vi "Dev List - New DTRow.vi"(7 "Row Index":i32, 8 "error in (no error)":errorcluster, 9 "Dev Data Lookup Table in":variant, 10 "DataGridView in":refnum<class "DataGridView.lvclass">, 11 "Controller UI in":refnum<class "Controller UI.lvclass">) -> (0 "error out":errorcluster, 1 "Dev Data Lookup Table in out":variant, 2 "DataGridView out":refnum<class "DataGridView.lvclass">)   [LabVIEW 2016, in "Controller UI.lvlib" / "Controller UI.lvclass"]
uses:
  <userlib>/Common Components/Controller UI/Controller UI.lvclass
  <userlib>/LabVIEWdotNetDataGrid/source/DataGridView/DataGridView.lvclass
  <userlib>/Common Components/Hardware/DevInfo/DevInfo Cluster Constant.ctl
  <userlib>/Common Components/Controller UI/Dev Variant Data.ctl
  <userlib>/Common Components/Hardware/DevInfo/DevInfo.lvclass
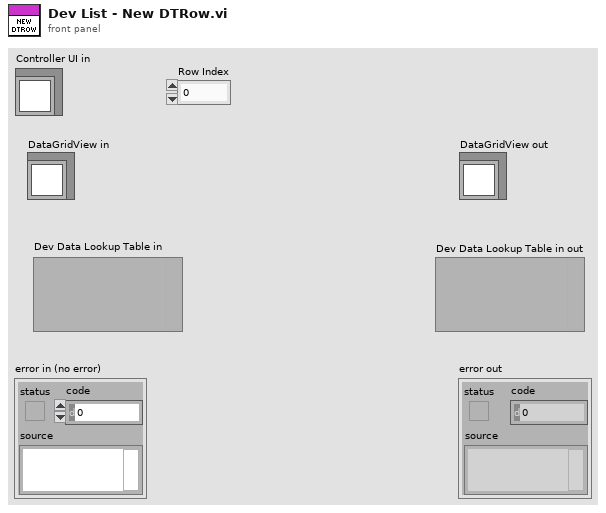
[diagram p1: front panel]
types:
  T1 = typedef "Controller UI.lvlib/Controller UI.lvclass/Dev Variant Data.ctl" = cluster{"Row Index":i32, "DevInfo Obj":refnum<class "DevInfo.lvclass">}
  T2 = typedef "Hardware.lvlib/DevInfo.lvclass/DevInfo Cluster Constant.ctl" = cluster{"GUID":string, "Check":string, "Checked-out":string, "Status":string, "Device":string, "Label":string, "COMM":string, "Sub-COMM":string, "COMM Settings":string}
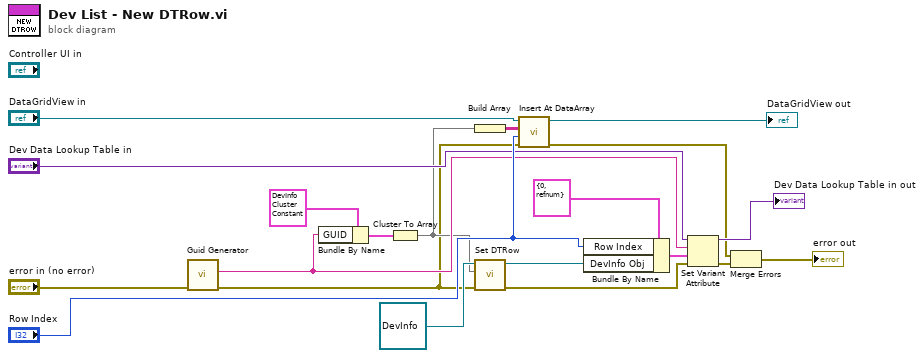
[diagram p0: block diagram]
diagram:
  n1 = call <vilib>:"Guid Generator.vi"("error in (no error)"="error in (no error)") -> ("error out"=w4:errorcluster, "GUID"=w11:string)  [unwired: 9 in]
  n2 = Bundle By Name(cluster=T2 {"GUID"="", "Check"="False", "Checked-out"="False", "Status"="off.png", "Device"="", "Label"="Enter a label", "COMM"="", "Sub-COMM"="", "COMM Settings"=""} ("Cluster"), "GUID"=w11) -> (w12:T2)
  n3 = Cluster To Array(cluster=w12) -> (array=w8:string[])
  n4 = Build Array(w8) -> (w14:string[][])
  n5 = call <userlib>:"Set DTRow.vi"("error in (no error)"=w4, "Dev Row Elements"=w8, "DevInfo in"=refnum<class "DevInfo.lvclass"> refnum ("DevInfo Obj")) -> ("error out"=w3:errorcluster, "DevInfo out"=w7:refnum<class "DevInfo.lvclass">)  [unwired: 7 in]
  n6 = call <userlib>:"Insert At DataArray.vi"("error in"=w4, "index"="Row Index", "Rows"=w14, "DataGridView in"="DataGridView in") -> ("error out"=w2:errorcluster, "DataGridView out"=→"DataGridView out":refnum<class "DataGridView.lvclass">)  [unwired: 6 in]
  n7 = Bundle By Name(cluster=T1 {"Row Index"=0, "DevInfo Obj"=refnum} ("Dev Data Lookup Table"), "Row Index"="Row Index", "DevInfo Obj"=w7) -> (w6:T1)
  n8 = Set Variant Attribute(Variant="Dev Data Lookup Table in", name=w11, value=w6, error in=w3) -> (Variant out=→"Dev Data Lookup Table in out":variant, error out=w1:errorcluster)  [unwired: 1 out]
  n9 = Merge Errors(w2, w1) -> (→"error out":errorcluster)
